vi "AlliGator Load Single Gate Image from Image Folder.vi"(6 "Action":T1, 8 "error in (no error)":errorcluster, 10 "File Info":variant, 11 "Gate Index":i32) -> (0 "error out":errorcluster, 1 "Data 2":sgl[][](array[numeric]), 3 "Data 1":sgl[][](array[numeric]))   [LabVIEW 2021, in "AlliGator Files.lvlib"]
doc: "Dynamically called VI to load a single gate image in a folder of gate images."
uses:
  AlliGator Files.lvlib
  HDF5/AlliGator FLI Image Stack Action.ctl
  AlliGator Image Folder Loading Information.ctl
  AlliGator RecSettings Metadata.ctl
  Files/Files.lvlib
  Image/Image.lvlib
  Strings/Strings.lvlib
  Error/Error.lvlib
  HDF5/AlliGator HDF5.lvlib
panel:
  # "see the AlliGator License on the block diagram (Ctrl+E or Window:Show Block Diagram)"
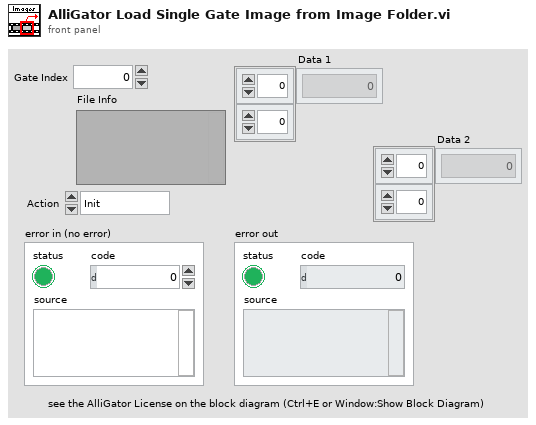
[diagram p1: front panel]
types:
  T1 = typedef "AlliGator HDF5.lvlib/AlliGator FLI Image Stack Action.ctl" = enum16{"Init", "Get Image", "Close"}
  T2 = typedef "AlliGator Files.lvlib/AlliGator Image Folder Loading Information.ctl" = cluster{"Image Folder":path, "Metadata":T3}
  T3 = typedef "AlliGator Files.lvlib/AlliGator RecSettings Metadata.ctl" = cluster{"Time Stamp (s)":dbl, "First Gate":dbl[unit], "Gate Step":dbl[unit], "# Gates":i32, "Gate Duration":dbl[unit], "Laser Period":dbl[unit], "Gate Image Integration":dbl[unit], "Date":timestamp, "V MCP":dbl[unit], "Binning":dbl}
  T4 = typedef "Image Type" = u32
  T5 = typedef "IMAQ Image.ctl" = refnum<image>
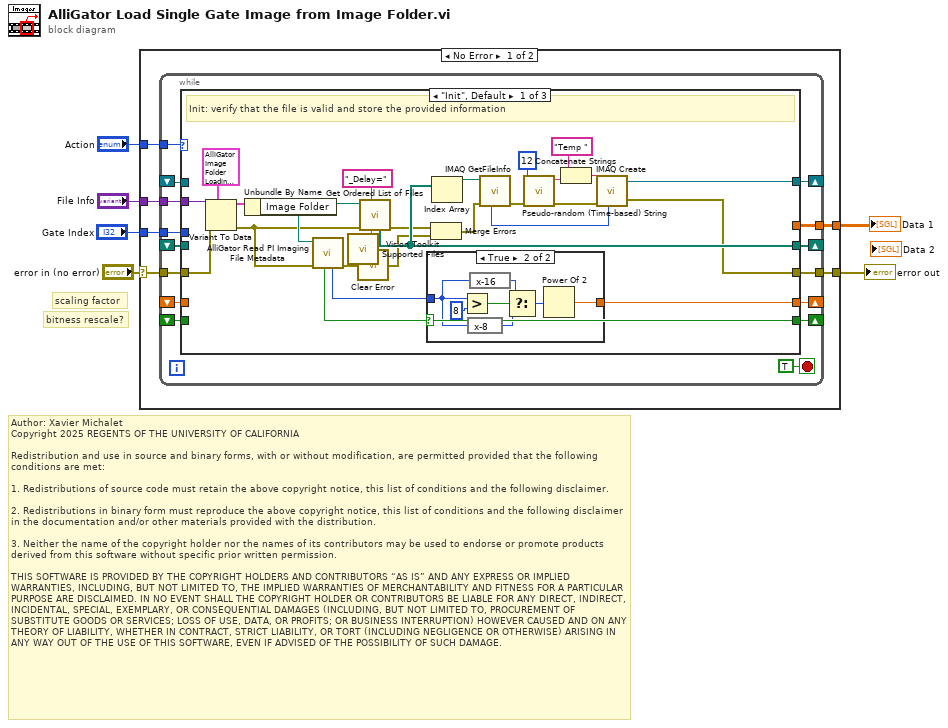
[diagram p0: block diagram]
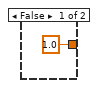
[diagram p2: hidden frame]
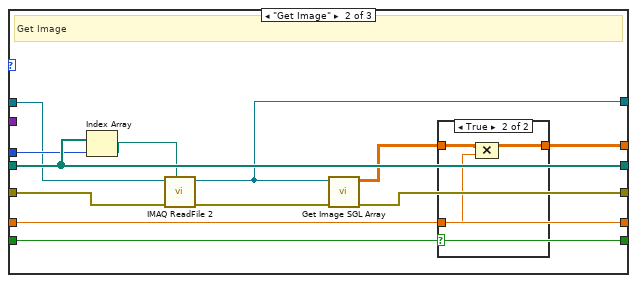
[diagram p3: hidden frame]
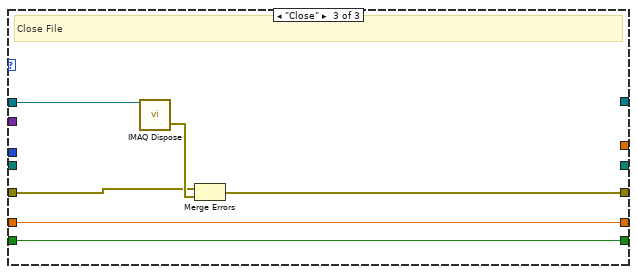
[diagram p5: hidden frame]
diagram:
  # "Author: Xavier Michalet\nCopyright 2025 REGENTS OF THE UNIVERSITY OF CALIFORNIA\n\nRedistribution and use in source and binary forms, with or without modification, are permitted provided that the following conditions are met:\n\n1. Redistributions of source code must retain the above copyright notice, this list of conditions and the following disclaimer.\n\n2. Redistributions in binary form must reproduce the above copyright notice, this list of conditions and the following disclaimer in the documentation and/or other materials provided with the distribution.\n\n3. Neither the name of the copyright holder nor the names of its contributors may be used to endorse or promote products derived from this software without specific prior written permission.\n\nTHIS SOFTWARE IS PROVIDED BY THE COPYRIGHT HOLDERS AND CONTRIBUTORS “AS IS” AND ANY EXPRESS OR IMPLIED WARRANTIES, INCLUDING, BUT NOT LIMITED TO, THE IMPLIED WARRANTIES OF MERCHANTABILITY AND FITNESS FOR A PARTICULAR PURPOSE ARE DISCLAIMED. IN NO EVENT SHALL THE COPYRIGHT HOLDER OR CONTRIBUTORS BE LIABLE FOR ANY DIRECT, INDIRECT, INCIDENTAL, SPECIAL, EXEMPLARY, OR CONSEQUENTIAL DAMAGES (INCLUDING, BUT NOT LIMITED TO, PROCUREMENT OF SUBSTITUTE GOODS OR SERVICES; LOSS OF USE, DATA, OR PROFITS; OR BUSINESS INTERRUPTION) HOWEVER CAUSED AND ON ANY THEORY OF LIABILITY, WHETHER IN CONTRACT, STRICT LIABILITY, OR TORT (INCLUDING NEGLIGENCE OR OTHERWISE) ARISING IN ANY WAY OUT OF THE USE OF THIS SOFTWARE, EVEN IF ADVISED OF THE POSSIBILITY OF SUCH DAMAGE."
  # "scaling factor"
  # "bitness rescale?"
  n1 = case shown="No Error" "error in (no error)" {
    selector: "error in (no error)" -> [w11 w84]
    tunnel: [w10 w84] -> w5
    tunnel: "Action" -> [w12 _]
    tunnel: "File Info" -> [w9 _]
    tunnel: "Gate Index" -> [w8 _]
    tunnel: [w7 _] -> w1
    frame No Error {
      n2 = while {
        tunnel: w12 -> [w26]
        tunnel: w11 -> [w25]
        tunnel: [w24] -> w10
        tunnel: w9 -> [w23]
        tunnel: w8 -> [w22]
        tunnel: [w21] -> w7
        shift-right: [w20] -> _
        shift-left: _ -> [w19]
        shift-right: [w18] -> _
        shift-left: _ -> [w17]
        shift-right: [w16] -> _
        shift-left: _ -> [w15]
        shift-right: [w14] -> _
        shift-left: _ -> [w13]
        stop <- TRUE stop-if-true
        n3 = case shown="\"Init\", Default" w26 {
          tunnel: w25 -> [w52 w69 w80]
          tunnel: [w42 w71 w81] -> w24
          tunnel: w23 -> [w53 _ _]
          tunnel: w22 -> [_ w72 _]
          tunnel: [_ w63 _] -> w21
          tunnel: [w47 w73 _] -> w20
          tunnel: w19 -> [_ w73 _]
          tunnel: [w43 w66 _] -> w18
          tunnel: w17 -> [_ w67 w83]
          tunnel: [w31 w62 w78] -> w16
          tunnel: w15 -> [_ w62 w78]
          tunnel: [w30 w65 w79] -> w14
          tunnel: w13 -> [_ w65 w79]
          frame "Init", Default {
            # "Init: verify that the file is valid and store the provided information"
            n4 = Variant To Data(error in=w52, type=T2 {"Image Folder"=path "", "Metadata"={"Time Stamp (s)"=0.0, "First Gate"=0.0, "Gate Step"=0.0, "# Gates"=0, "Gate Duration"=0.0, "Laser Period"=0.0, "Gate Image Integration"=0.0, "Date"=timestamp(0 s since 1904-01-01), "V MCP"=0.0, "Binning"=0.0}} ("Image Folder Loading Information"), Variant=w53) -> (data=w48:T2, error out=w34:errorcluster)
            n5 = Unbundle By Name(w48) -> ("Image Folder"=w35:path)
            n6 = call "AlliGator Read PI Imaging File Metadata.vi"("error in"=w34, "Image Folder"=w35) -> ("error out"=w29:errorcluster, "bitness"=w32:i32, "Correct bit shift"=w30:bool)  [unwired: 5 in, 2 out]
            n7 = call "Vision Toolkit Supported Files.vi"() -> ("Pattern String"=w50:string)  [unwired: 7 in, 1 out]
            n8 = call "Clear Error.vi"("Error In"=w29) -> ("no Error Out"=w28:errorcluster)  [unwired: 8 in]
            n9 = call "Get Ordered List of Files.vi"("pattern"=w50, "Split string"="_Delay=", "Error In"=w34, "Folder Path"=w35) -> ("Error Out"=w45:errorcluster, "Ordered File Paths"=w47:path[])  [unwired: 4 in, 2 out]
            n10 = case shown="True" w30 {
              tunnel: w32 -> [_ w57]
              tunnel: [1.0 w55] -> w31
              frame False {
              }
              frame True {
                n11 = Greater?(x=w57, y=8) -> (0:w60:bool)
                n12 = expression code="x-8"(w57) -> (w59:i32)
                n13 = expression code="x-16"(w57) -> (w56:i32)
                n14 = Select(t=w56, s=w60, f=w59) -> (s? t:f=w58:i32)
                n15 = Power Of 2(x=w58) -> (2^x=w55:dbl)
              }
            }
            n16 = Merge Errors(w45, w28) -> (w33:errorcluster)
            n17 = Index Array(array=w47) -> (element=w46:path)  [unwired: 1 in]
            n18 = call "IMAQ GetFileInfo"("error in (no error)"=w33, "File Path"=w46) -> ("error out"=w40:errorcluster, "Image Type"=w44:T4)  [unwired: 3 in, 5 out]
            n19 = call "Pseudo-random (Time-based) String.vi"("Error In"=w40, "Length (10)"=u32 12) -> ("Error Out"=w39:errorcluster, "result string"=w41:string)  [unwired: 8 in]
            n20 = Concatenate Strings("Temp " ("string"), w41) -> (w38:string)
            n21 = call "IMAQ Create"("Image Name"=w38, "Image Type"=w44, "error in (no error)"=w39) -> ("New Image"=w43:T5, "error out"=w42:errorcluster)  [unwired: 2 in]
          }
          frame "Get Image" {
            # "Get Image"
            n22 = Index Array(array=w73, index=w72) -> (element=w70:path)
            n23 = call "IMAQ ReadFile 2"("File Path"=w70, "error in (no error)"=w69, "Image"=w67) -> ("error out"=w68:errorcluster, "Image Out"=w66:T5)  [unwired: 4 in, 3 out]
            n24 = call "Get Image SGL Array.vi"("error in (no error)"=w68, "Refnum in"=w66) -> ("error out"=w71:errorcluster, "Pixel Array"=w64:sgl[][])  [unwired: 8 in]
            n25 = case shown="True" w65 {
              tunnel: w64 -> [w74 w77]
              tunnel: [w74 w75] -> w63
              tunnel: w62 -> [_ w76]
              frame False {
              }
              frame True {
                n26 = Compound Arithmetic op=MULTIPLY(w77, w76) -> (w75:dbl[][])
              }
            }
          }
          frame "Close" {
            # "Close File"
            n27 = call "IMAQ Dispose"("Image"=w83) -> ("error out"=w82:errorcluster)  [unwired: 5 in]
            n28 = Merge Errors(w80, w82) -> (w81:errorcluster)
          }
        }
      }
    }
    frame Error {
    }
  }
  "Data 1" <- w1
  "error out" <- w5
